vi "Display Artist Library.vi"(8 "error in (no error)":errorcluster, 10 "MusicLibrary":refnum<class "MusicLibrary.lvclass">, 11 "SongBrowserActor in":refnum<class "SongBrowserActor.lvclass">) -> (0 "error out":errorcluster, 3 "SongBrowserActor out":refnum<class "SongBrowserActor.lvclass">)   [LabVIEW 2015, in "SongBrowserActor.lvlib" / "SongBrowserActor.lvclass"]
uses:
  SongBrowserActor.lvclass
  file/MusicElement/MusicElementLibrary/MusicLibrary/MusicLibrary.lvclass
  SongBrowserActor.lvclass/SongBrowserActor.ctl
  builds/xctls/Artist Browser/Artist Browser.lvlibp/app/xctls/Artist Browser/Artist Browser.xctl
  file/MusicElement/MusicElementLibrary/MusicElementLibrary.lvclass
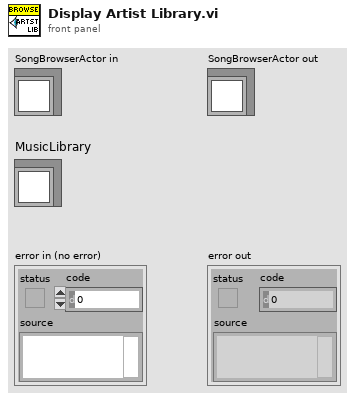
[diagram p1: front panel]
types:
  T1 = typedef "Music Library Element Display.ctl" = cluster{"Name":string, "Details":string, "Duration (s)":T2, "Click":bool}
  T2 = typedef "Song.lvclass/Song Duration.ctl" = timestamp
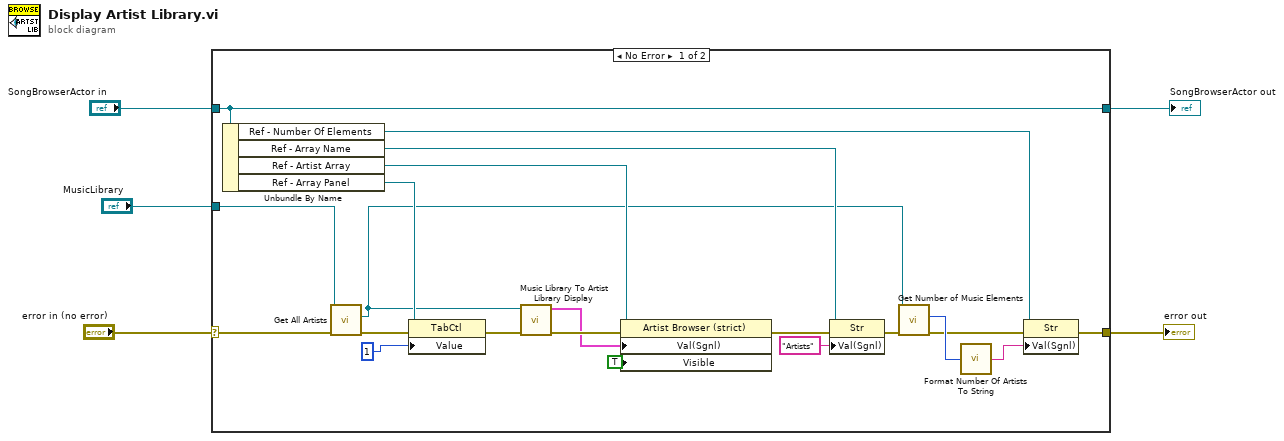
[diagram p0: block diagram]
diagram:
  n1 = case shown="No Error" "error in (no error)" {
    selector: "error in (no error)" -> [w12 w28]
    tunnel: [w19 w28] -> w4
    tunnel: [w26 w27] -> w2
    tunnel: "SongBrowserActor in" -> [w26 w27]
    tunnel: "MusicLibrary" -> [w11 _]
    frame No Error {
      n2 = Unbundle By Name(w26) -> ("Ref - Number Of Elements"=w20:refnum<vi>, "Ref - Array Name"=w22:refnum<vi>, "Ref - Artist Array"=w25:refnum<vi>, "Ref - Array Panel"=w14:refnum<vi>)
      n3 = call "Get All Artists.vi"("error in (no error)"=w12, "MusicLibrary in"=w11) -> ("error out"=w10:errorcluster, "Artist Library"=w8:refnum<class "MusicLibrary.lvclass">)  [unwired: 7 in, 1 out]
      n4 = property class="TabCtl"(reference=w14, error in=w10, "Value"=1) -> (error out=w13:errorcluster)  [unwired: 1 out]
      n5 = call "Music Library To Artist Library Display.vi"("error in (no error)"=w13, "Artist Library"=w8) -> ("error out"=w18:errorcluster, "Music Library Display Array"=w17:T1[])  [unwired: 8 in]
      n6 = property class="Artist Browser (strict)"(reference=w25, error in=w18, "Val(Sgnl)"=w17, "Visible"=TRUE) -> (error out=w23:errorcluster)  [unwired: 1 out]
      n7 = property class="Str"(reference=w22, error in=w23, "Val(Sgnl)"="Artists" ("Value (Signaling)")) -> (error out=w9:errorcluster)  [unwired: 1 out]
      n8 = call "Get Number of Music Elements.vi"("error in (no error)"=w9, "MusicElementLibrary in"=w8) -> ("error out"=w6:errorcluster, "Size"=w7:i32)  [unwired: 7 in, 1 out]
      n9 = call "Format Number Of Artists To String.vi"("Number Of Songs"=w7) -> ("Formatted"=w16:string)
      n10 = property class="Str"(reference=w20, error in=w6, "Val(Sgnl)"=w16) -> (error out=w19:errorcluster)  [unwired: 1 out]
    }
    frame Error {
    }
  }
  "error out" <- w4
  "SongBrowserActor out" <- w2
